vi "Read Cells.vi"(8 "error in (no error)":errorcluster, 11 "PAS in":refnum<class "PAS.lvclass">) -> (0 "error out":errorcluster, 2 "Cells":refnum<class "PAS Cell.lvclass">[](array[class]), 3 "PAS out":refnum<class "PAS.lvclass">)   [LabVIEW 2016, in "PAS Library.lvlib" / "PAS.lvclass"]
uses:
  PAS.lvclass
  Cell/PAS Cell.lvclass
  PAS.lvclass/PAS.ctl
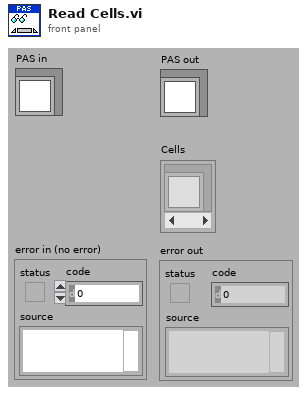
[diagram p1: front panel]
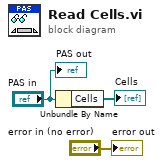
[diagram p0: block diagram]
diagram:
  n1 = Unbundle By Name("PAS in") -> ("Cells"=→"Cells":refnum<class "PAS Cell.lvclass">[])
  "error out" <- "error in (no error)"
  "PAS out" <- "PAS in"
